vi "Description.vi"(8 "error in (no error)":errorcluster, 11 "Tolerant Numeric Input Comparator in":refnum<class "Tolerant Numeric Input Comparator.lvclass">) -> (0 "error out":errorcluster, 2 "Description":string)   [LabVIEW 2020, in "Tolerant Numeric Input Comparator.lvclass"]
uses:
  Tolerant Numeric Input Comparator.lvclass
  Tolerant Numeric Input Comparator.lvclass/Tolerant Numeric Input Comparator.ctl
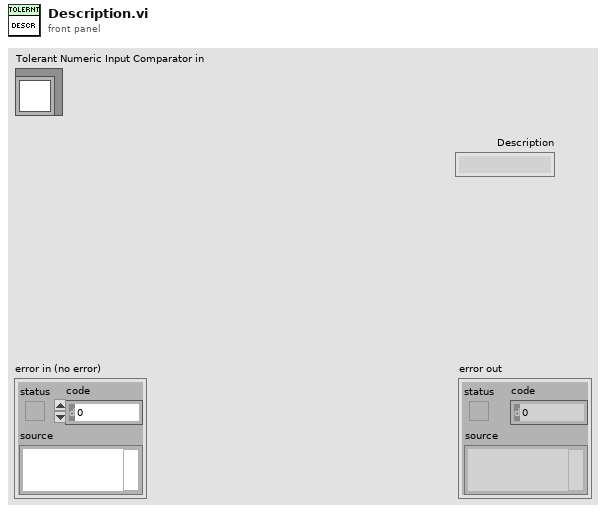
[diagram p1: front panel]
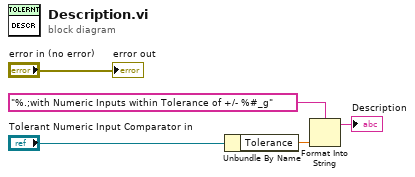
[diagram p0: block diagram]
diagram:
  n1 = Unbundle By Name("Tolerant Numeric Input Comparator in") -> ("Tolerance"=w2:dbl)
  n2 = Format Into String(format string="%.;with Numeric Inputs within Tolerance of +/- %#_g" ("Description"), w2) -> (resulting string=→"Description":string)  [unwired: 2 in, 1 out]
  "error out" <- "error in (no error)"
